vi "PathPlanning.vi"(7 "Goal":cluster{"X":i16, "Y":i16}, 8 "error in":errorcluster, 9 "Corners":cluster{"Col":i16, "Row":i16}[](array[cluster]), 10 "Map":i8[][](array[numeric]), 11 "Robot in map":cluster{"Col":i16, "Row":i16}) -> (0 "error out":errorcluster, 2 "PathPoints":T1)   [LabVIEW 2009, in "Main.lvlib"]
doc: "Main path planning algorithm. Calculates path to the goal from map information."
uses:
  Main.lvlib
  Navigation/Nav_CordinateArray.ctl
  Navigation.lvlib
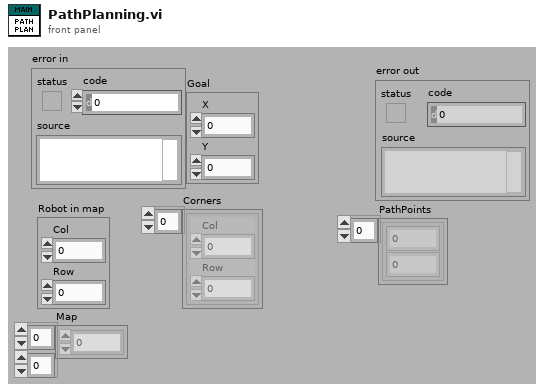
[diagram p1: front panel]
types:
  T1 = typedef "Navigation.lvlib/Nav_CordinateArray.ctl" = cluster{"X position":dbl, "Y position":dbl}[]
  T2 = cluster{"Robot":cluster{"X":i16, "Y":i16, "Bearing":dbl}, "Map":i8[][], "Goal":cluster{"X":i16, "Y":i16}, "Corners":cluster{"X":i16, "Y":i16}[]}
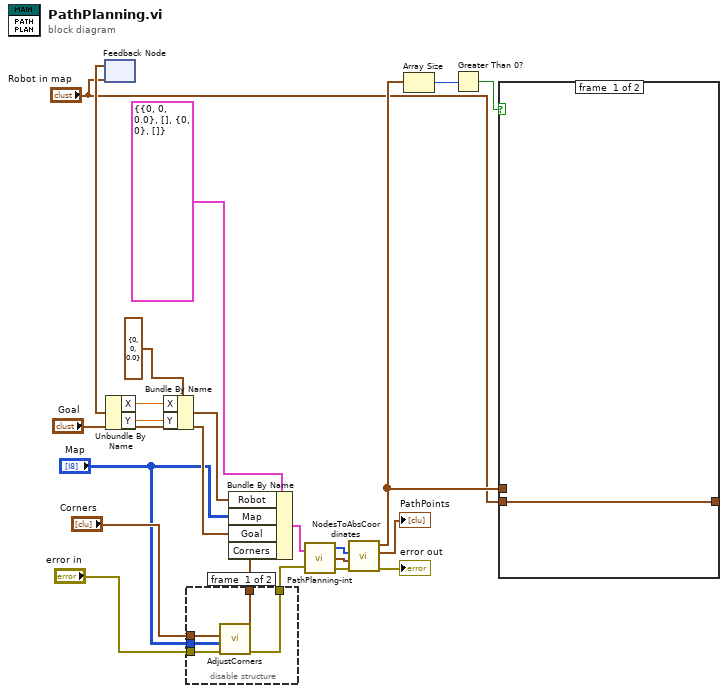
[diagram p0: block diagram]
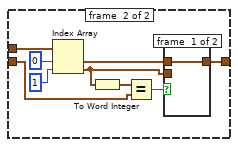
[diagram p3: hidden frame]
diagram:
  n1 = feedback #1("Robot in map") -> (w7:cluster{"X":dbl, "Y":dbl})
  n2 = Unbundle By Name(w7) -> ("X"=w2:dbl, "Y"=w1:dbl)
  n3 = Bundle By Name(cluster=cluster{"X":i16, "Y":i16, "Bearing":dbl} {"X"=0, "Y"=0, "Bearing"=0.0} ("Robot"), "X"=w2, "Y"=w1) -> (w8:cluster{"X":i16, "Y":i16, "Bearing":dbl})
  n4 = disable-structure shown="Enabled" {
    disable-tunnel: "error in" -> [w28 w29]
    disable-tunnel: [w27 w29] -> w14
    disable-tunnel: "Corners" -> [w26 w30]
    disable-tunnel: [w25 w30] -> w12
    disable-tunnel: "Map" -> [w24 _]
    frame #0 {
      n5 = call "AdjustCorners.vi"("error in"=w28, "Map"=w24, "Corners"=w26) -> ("error out"=w27:errorcluster, "Corners out"=w25:cluster{"Col":i16, "Row":i16}[])  [unwired: 7 in]
    }
    frame #1 {
    }
  }
  n6 = Bundle By Name(cluster=T2 {"Robot"={"X"=0, "Y"=0, "Bearing"=0.0}, "Map"=[], "Goal"={"X"=0, "Y"=0}, "Corners"=[]} ("Map&Nodes"), "Robot"=w8, "Map"="Map", "Goal"="Goal", "Corners"=w12) -> (w17:T2)
  n7 = call "PathPlanning-int.vi"("Map&Nodes"=w17, "error in (no error)"=w14) -> ("Path"=w19:i32[], "Coordinates"=w20:cluster{"X":dbl, "Y":dbl}[], "error out"=w21:errorcluster)
  n8 = call "NodesToAbsCoordinates.vi"("error in"=w21, "Coordinates"=w20, "Path"=w19) -> ("error out"=→"error out":errorcluster, "Points output"=→"PathPoints":T1, "Map_Points"=w6:cluster{"X":dbl, "Y":dbl}[])  [unwired: 6 in]
  n9 = Array Size(array=w6) -> (size(s)=w5:i32)
  n10 = Greater Than 0?(x=w5) -> (x > 0?=w4:bool)
  n11 = case shown="True" w4 {
    tunnel: [w31 w40] -> w9
    tunnel: w6 -> [_ w37]
    tunnel: "Robot in map" -> [w31 w35]
    frame #0 {
    }
    frame #1 {
      n12 = Index Array(array=w37, index #1=0 ("index"), index #2=1 ("index")) -> (element #1=w36:cluster{"X":dbl, "Y":dbl}, element #2=w34:cluster{"X":dbl, "Y":dbl})
      n13 = To Word Integer(number=w34) -> (16bit integer=w33:cluster{"X":i16, "Y":i16})
      n14 = Equal?(x=w33, y=w35) -> (x = y?=w32:bool)
      n15 = case shown="True" w32 {
        tunnel: [w41 w42] -> w40
        tunnel: w36 -> [w41 _]
        tunnel: w34 -> [_ w42]
        frame #0 {
        }
        frame #1 {
        }
      }
    }
  }
